vi "Large Signal Bench GUI.vi"() -> ()   [LabVIEW 2020, in "NI USB-6501.lvclass"]
uses:
  NI USB-6501.lvclass
  Path Control/Measurements Specific Paths.ctl
  <vilib>/DAQmx/read.llb/DAQmx Read (Digital Bool 1Line 1Point).vi
  <vilib>/DAQmx/write.llb/DAQmx Write (Digital Bool 1Line 1Point).vi
  <vilib>/DAQmx/miscellaneous.llb/DAQmx Fill In Error Info.vi
  Path Control/PathControl.lvclass
panel:
  out "error out":errorcluster
  in  "SG1 Switch":T1
  out "PA2 thermal shut-off indicator":bool
  in  "PA2 Power":bool
  in  "SA input":enum32{"Radio Selection 1", "Radio Selection 2"}(radio)
  in  "Exit":bool
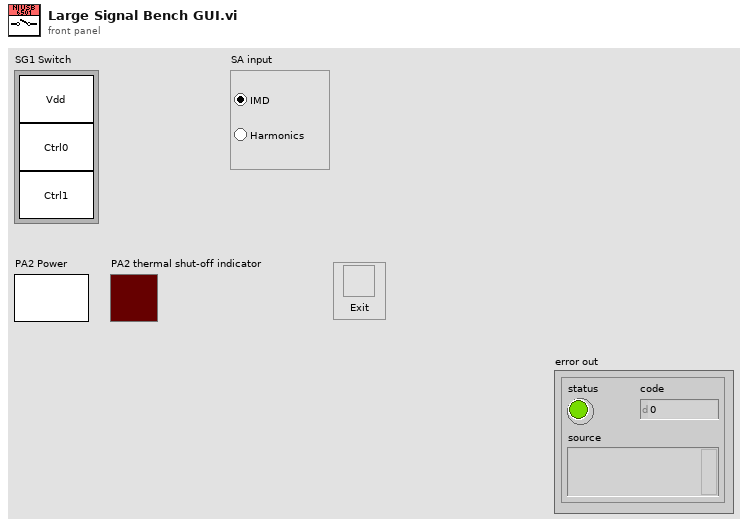
[diagram p1: front panel]
types:
  T1 = cluster{"SG1 switch Vdd":bool, "SG1 switch Ctrl0":bool, "SG1 switch Ctrl1":bool}
  T2 = typedef "PathControl.lvclass/Measurements Specific Paths.ctl" = enum16{"No calibration", "Harmonics", "IMD", "S Parameter", "AM-AM", "MCCW-ACLR", "DC", "LCR", "Power Meter GUI", "RF Power"}
  T3 = enum8{"Enabled", "Disabled", "Disabled and Grayed Out"}
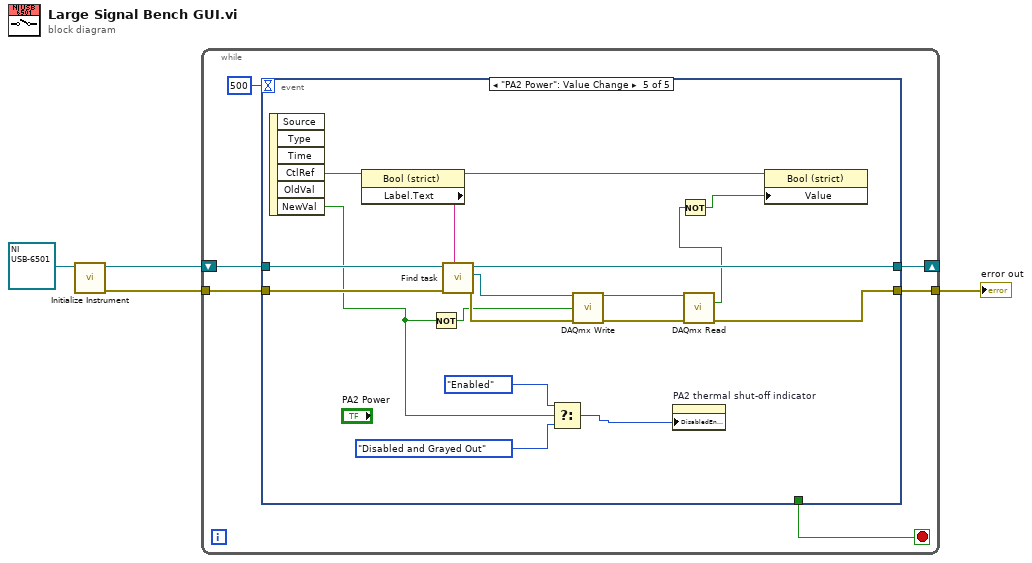
[diagram p0: block diagram]
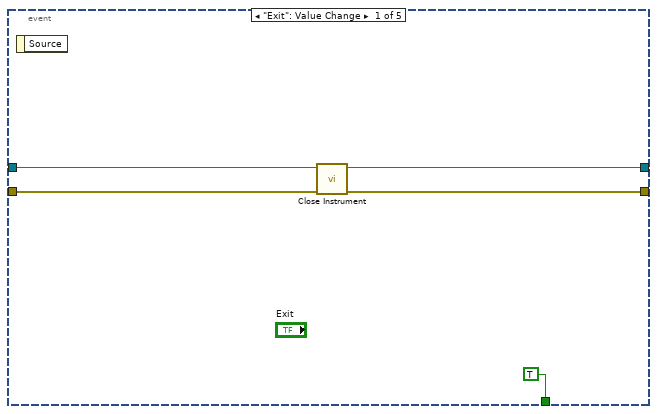
[diagram p2: hidden frame]
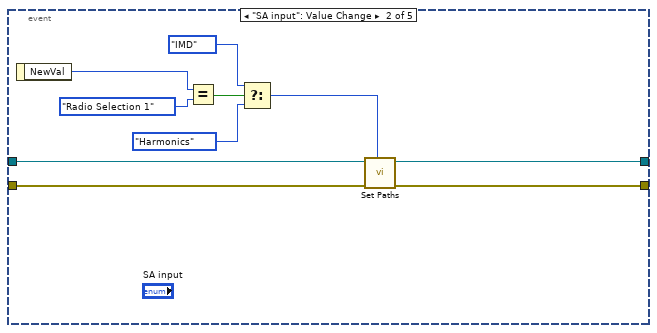
[diagram p3: hidden frame]
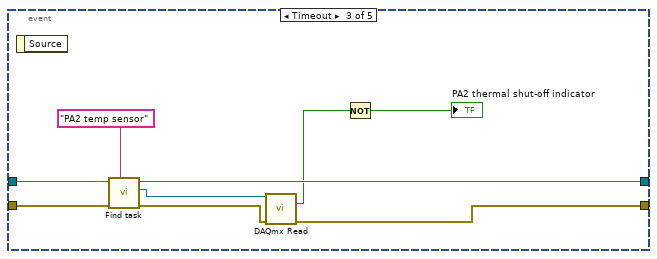
[diagram p4: hidden frame]
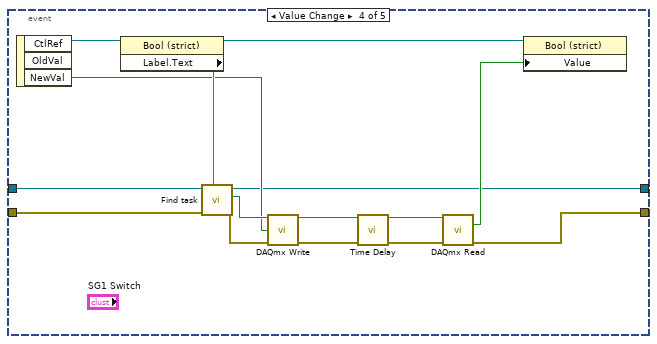
[diagram p5: hidden frame]
diagram:
  n1 = call-dynamic "Initialize Instrument.vi"("NI USB-6501 in"=refnum<class "NI USB-6501.lvclass"> refnum) -> ("error out"=w2:errorcluster, "NI USB-6501 out"=w1:refnum<class "NI USB-6501.lvclass">)  [unwired: 9 in]
  n2 = while {
    tunnel: w2 -> [w10]
    tunnel: [w8] -> w3
    shift-right: [w7] -> _
    shift-left: w1 -> [w5]
    stop <- w9 stop-if-true
    n3 = event shown="[4] \"PA2 Power\": Value Change" {
      selector: _ -> [_ _ _ _ _]
      dyn-events: _ -> [_ _ _ _ _]
      timeout: 500 -> [_ _ _ _ _]
      tunnel: w5 -> [w15 w25 w34 w48 w59]
      tunnel: w10 -> [w14 w24 w33 w47 w60]
      tunnel: [TRUE _ _ _ _] -> w9
      tunnel: [w12 w23 w29 w38 w58] -> w8
      tunnel: [w11 w22 w32 w37 w57] -> w7
      event "Exit": Value Change {
        n4 = event-data() -> ()  [unwired: 1 in, 1 out]
        n5 = call-dynamic "Close Instrument.vi"("error in (no error)"=w14, "NI USB-6501 in"=w15) -> ("error out"=w12:errorcluster, "NI USB-6501 out"=w11:refnum<class "NI USB-6501.lvclass">)  [unwired: 8 in]
      }
      event "SA input": Value Change {
        n6 = event-data() -> ("NewVal"=w20:enum32{"Radio Selection 1", "Radio Selection 2"})  [unwired: 1 in]
        n7 = Equal?(x=w20, y=enum32{"Radio Selection 1", "Radio Selection 2"}."Radio Selection 1" ("NewVal")) -> (x = y?=w18:bool)
        n8 = Select(t=Measurements_Specific_Paths."IMD" ("Measurement specfic paths"), s=w18, f=Measurements_Specific_Paths."Harmonics" ("Measurement specfic paths")) -> (s? t:f=w16:T2)
        n9 = call-dynamic "Set Paths.vi"("Measurement specific paths"=w16, "error in (no error)"=w24, "NI USB-6501 in"=w25) -> ("error out"=w23:errorcluster, "NI USB-6501 out"=w22:refnum<class "NI USB-6501.lvclass">)  [unwired: 7 in]
      }
      event Timeout {
        n10 = event-data() -> ()  [unwired: 1 in, 1 out]
        n11 = call "Find task.vi"("Function"="PA2 temp sensor", "error in (no error)"=w33, "NI USB-6501 in"=w34) -> ("error out"=w31:errorcluster, "Task"=w30:refnum<k21>, "NI USB-6501 out"=w32:refnum<class "NI USB-6501.lvclass">)  [unwired: 6 in]
        n12 = call-poly <vilib>:"DAQmx Read.vi"("task/channels in"=w30, "error in"=w31) -> ("data"=w27:bool, "error out"=w29:errorcluster)  [unwired: 11 in, 1 out]
        n13 = Not(x=w27) -> (.not. x?=→"PA2 thermal shut-off indicator":bool)
      }
      event "SG1 Switch.SG1 switch Vdd", "SG1 Switch.SG1 switch Ctrl0", "SG1 Switch.SG1 switch Ctrl1": Value Change {
        n14 = event-data() -> ("CtlRef"=w46:refnum<vi>, "NewVal"=w41:bool)  [unwired: 1 in, 1 out]
        n15 = property class="Bool (strict)"(reference=w46) -> (reference out=w40:refnum<vi>, "Label.Text"=w45:string)  [unwired: 1 in, 1 out]
        n16 = call "Find task.vi"("Function"=w45, "error in (no error)"=w47, "NI USB-6501 in"=w48) -> ("error out"=w42:errorcluster, "Task"=w43:refnum<k21>, "NI USB-6501 out"=w37:refnum<class "NI USB-6501.lvclass">)  [unwired: 6 in]
        n17 = call-poly <vilib>:"DAQmx Write.vi"("task/channels in"=w43, "data"=w41, "error in"=w42) -> ("task out"=w44:refnum<k21>, "error out"=w36:errorcluster)  [unwired: 10 in, 1 out]
        n18 = call "Time Delay"("error in (no error)"=w36) -> ("error out"=w35:errorcluster)  [unwired: 10 in]
        n19 = call-poly <vilib>:"DAQmx Read.vi"("task/channels in"=w44, "error in"=w35) -> ("data"=w39:bool, "error out"=w38:errorcluster)  [unwired: 11 in, 1 out]
        n20 = property class="Bool (strict)"(reference=w40, "Value"=w39) -> ()  [unwired: 1 in, 2 out]
      }
      event "PA2 Power": Value Change {
        n21 = event-data() -> ("CtlRef"=w56:refnum<vi>, "NewVal"=w52:bool)  [unwired: 1 in, 4 out]
        n22 = property class="Bool (strict)"(reference=w56) -> (reference out=w61:refnum<vi>, "Label.Text"=w66:string)  [unwired: 1 in, 1 out]
        n23 = Not(x=w52) -> (.not. x?=w51:bool)
        n24 = call "Find task.vi"("Function"=w66, "error in (no error)"=w60, "NI USB-6501 in"=w59) -> ("error out"=w62:errorcluster, "Task"=w63:refnum<k21>, "NI USB-6501 out"=w57:refnum<class "NI USB-6501.lvclass">)  [unwired: 6 in]
        n25 = Select(t=T3."Enabled" ("Disabled"), s=w52, f=T3."Disabled and Grayed Out" ("Disabled")) -> (s? t:f=w53:T3)
        n26 = call-poly <vilib>:"DAQmx Write.vi"("task/channels in"=w63, "data"=w51, "error in"=w62) -> ("task out"=w65:refnum<k21>, "error out"=w64:errorcluster)  [unwired: 10 in, 1 out]
        n27 = property on="PA2 thermal shut-off indicator" class="Bool (strict)"("DisabledEnum"=w53) -> ()  [unwired: 2 in, 2 out]
        n28 = call-poly <vilib>:"DAQmx Read.vi"("task/channels in"=w65, "error in"=w64) -> ("data"=w50:bool, "error out"=w58:errorcluster)  [unwired: 11 in, 1 out]
        n29 = Not(x=w50) -> (.not. x?=w49:bool)
        n30 = property class="Bool (strict)"(reference=w61, "Value"=w49) -> ()  [unwired: 1 in, 2 out]
      }
    }
  }
  "error out" <- w3
